vi "Ping.vi"(11 "Host IP Address":string="127.0.0.1") -> (0 "error out":errorcluster, 2 "Status":i32(ring) items=["Success"=0, "DestinationNetworkUnreachable"=11002, "DestinationHostUnreachable"=11003, "DestinationProhibited, DestinationProtocolUnreachable"=11004, "DestinationPortUnreachable"=11005, "NoResources"=11006, "BadOption"=11007, "HardwareError"=11008, "PacketTooBig"=11009, "TimedOut"=11010, "BadRoute"=11012, "TtlExpired"=11013, "TtlReassemblyTimeExceeded"=11014, "ParameterProblem"=11015, "SourceQuench"=11016, "BadDestination"=11018, "DestinationUnreachable"=11040, "TimeExceeded"=11041, "BadHeader"=11042, "UnrecognizedNextHeader"=11043, "IcmpError"=11044, "DestinationScopeMismatch"=11045, "Unknown"=-1], 3 "success":bool)   [LabVIEW 2016]
panel:
  out "Execution Time":u32
  in  "timeout":i32=100
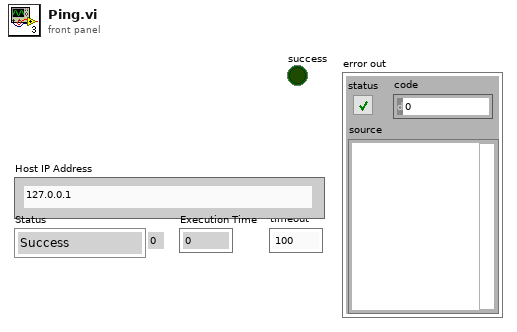
[diagram p1: front panel]
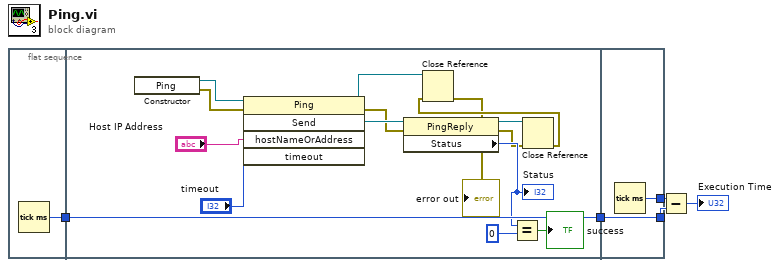
[diagram p0: block diagram]
diagram:
  n1 = flat-sequence {
    tunnel: [w6] -> w5
    tunnel: w5 -> [w15]
    tunnel: [w15] -> w4
    tunnel: [w23] -> w3
    tunnel: w4 -> [w22]
    tunnel: [w22] -> w2
    frame #0 {
      n2 = Tick Count (ms)() -> (millisecond timer value=w6:u32)
    }
    frame #1 {
      n3 = constructor class="Ping"() -> (reference out=w18:refnum<k24>, error out=w11:errorcluster)  [unwired: 3 in, 1 out]
      n4 = invoke class="Ping" method="Send"(reference=w18, error in=w11, "hostNameOrAddress"="Host IP Address", "timeout"="timeout") -> (reference out=w16:refnum<k24>, error out=w10:errorcluster, "Send"=w20:refnum<k24>)  [unwired: 1 in, 2 out]
      n5 = property class="PingReply"(reference=w20, error in=w10) -> (reference out=w17:refnum<k24>, error out=w9:errorcluster, "Status"=w14:i32)
      "Status" <- w14
      n6 = Equal?(x=w14, y=0) -> (x = y?=→"success":bool)
      n7 = Close Reference(reference=w17, error in (no error)=w9) -> (error out=w8:errorcluster)
      n8 = Close Reference(reference=w16, error in (no error)=w8) -> (error out=→"error out":errorcluster)
    }
    frame #2 {
      n9 = Tick Count (ms)() -> (millisecond timer value=w23:u32)
    }
  }
  n10 = Subtract(x=w3, y=w2) -> (x-y=→"Execution Time":u32)
